vi "A33ConfigureFSweep_py.vi"(1 "Enable Frequency Sweep (T:Enable)":bool=TRUE, 2 "Sweep Time (1.0 Seconds)":dbl=1.0 format="%#.6g", 5 "Channel (1: Channel1)":i32(ring)=1 items=["Channel1"=1, "Channel2"=2], 7 "Sweep Spacing (0: Linear)":i32(ring) items=["Linear", "Logarithmic"], 9 "Start Frequency (1.0 uHz)":dbl=1e-06 format="%#.12g", 12 "Stop  Frequency  (1000.0 Hz)":dbl=1000.0 format="%#.12g", 13 "Hold Time (0 Seconds)":dbl format="%#.6g", 14 "Return Time (0 Seconds)":dbl format="%#.6g") -> ()   [LabVIEW 2022 SP3]
doc: "Configures and enables a frequency sweep. In the frequency sweep mode, the function generator steps from the start frequency to the stop frequency at a sweep rate."
uses:
  <vilib>/addons/zeromq/zmq_socket.lvclass
panel:
  out "Standalone":bool
  out "socket out":refnum<class "zmq_socket.lvclass">
  in  "socket in":refnum<class "zmq_socket.lvclass">
  out "error out 2":errorcluster
  out "resulting string":string
  in  "Instrument":string
  in  "error in (no error) 2":errorcluster
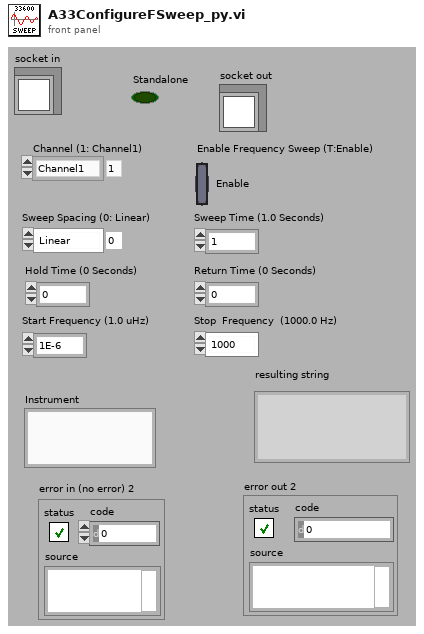
[diagram p1: front panel]
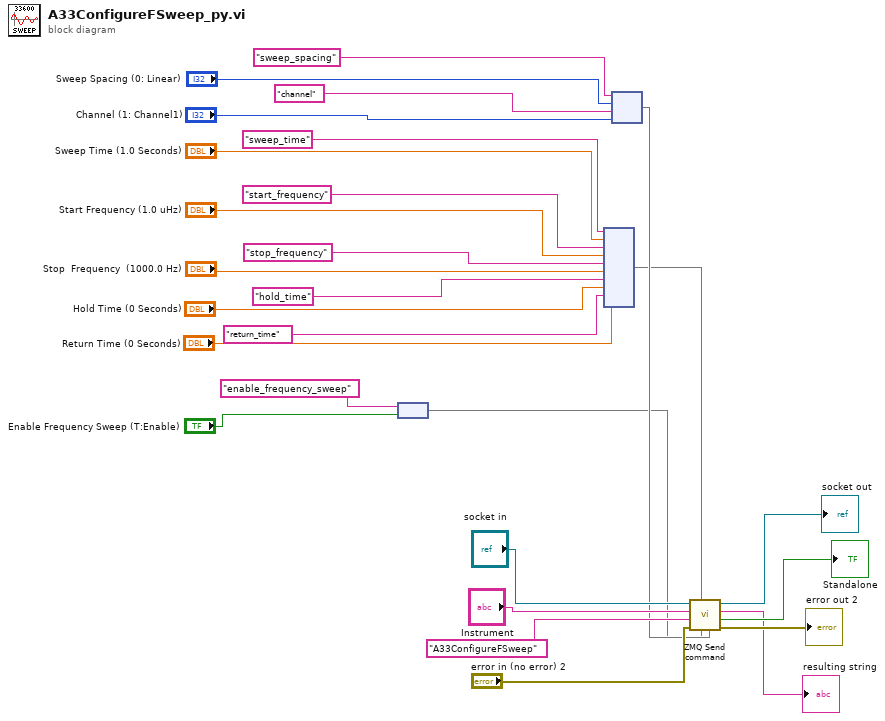
[diagram p0: block diagram]
diagram:
  n1 = node("enable_frequency_sweep" ("key"), "Enable Frequency Sweep (T:Enable)") -> (w3:map{string, bool})
  n2 = node("sweep_time" ("key"), "Sweep Time (1.0 Seconds)", "start_frequency" ("key"), "Start Frequency (1.0 uHz)", "stop_frequency" ("key"), "Stop  Frequency  (1000.0 Hz)", "hold_time" ("key"), "Hold Time (0 Seconds)", "return_time" ("key"), "Return Time (0 Seconds)") -> (w14:map{string, dbl})
  n3 = node("sweep_spacing" ("key"), "Sweep Spacing (0: Linear)", "channel" ("key"), "Channel (1: Channel1)") -> (w15:map{string, i32})
  n4 = call "ZMQ Send command.vi"("Int args"=w15, "Bool args"=w3, "DBL args"=w14, "error in"="error in (no error) 2", "Command"="A33ConfigureFSweep", "Instrument"="Instrument", "socket in"="socket in") -> ("error out"=→"error out 2":errorcluster, "Standalone"=→"Standalone":bool, "Recieved message"=→"resulting string":string, "socket out"=→"socket out":refnum<class "zmq_socket.lvclass">)  [unwired: 1 in]
